vi "Construct PDU.vi"(8 "error in":errorcluster, 10 "data":u8[](array[numeric]), 11 "Function":T1 items=["Read Discrete Inputs"=2, "Read Coils"=1, "Write Single Coil"=5, "Write Multiple Coils"=15, "Read Input Register"=4, "Read Holding Registers"=3, "Write Single Register"=6, "Write Multiple Registers"=16, "Read/Write Multiple Registers"=23, "Mask Write Register"=22, "Read FIFO Queue"=24, "Read File Record"=20, "Write File Record"=21, "Read Exception Status"=7, "Diagnostic"=8, "Get Com Event Counter"=11, "Get Com Event Log"=12, "Report Slave ID"=17, "Read Device Identification"=43]) -> (0 "error out":errorcluster, 3 "modbus data unit out":refnum<class "Modbus Data Unit.lvclass">)   [LabVIEW 2012, in "Modbus Data Unit.lvclass"]
uses:
  Modbus Data Unit.lvclass
  Function.ctl
  Modbus Data Unit.lvclass/Modbus Data Unit.ctl
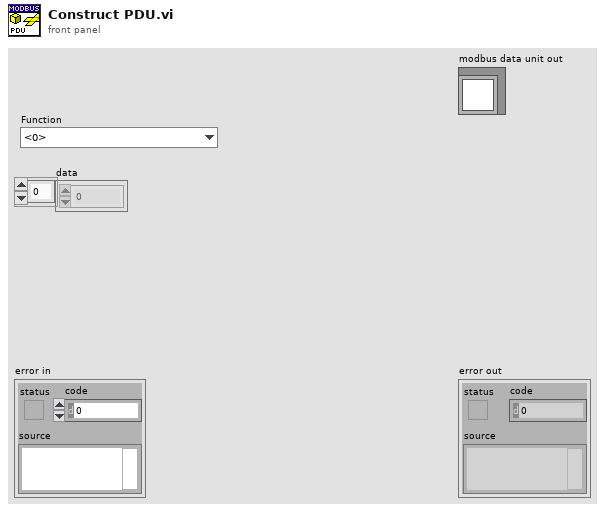
[diagram p1: front panel]
types:
  T1 = typedef "Modbus Data Unit.lvclass/Function.ctl" = u8
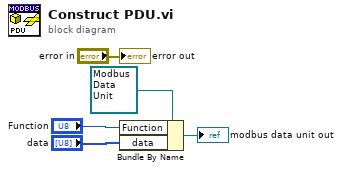
[diagram p0: block diagram]
diagram:
  n1 = Bundle By Name(cluster=refnum<class "Modbus Data Unit.lvclass"> refnum ("modbus data unit"), "Function"="Function", "data"="data") -> (→"modbus data unit out":refnum<class "Modbus Data Unit.lvclass">)
  "error out" <- "error in"
